vi "Initialize MeasurementLink Session.vi"(7 "remote connection options":T2, 8 "error in (no error)":errorcluster, 9 "initialize and close session behavior":T1, 10 "session initialization parameters":T3, 11 "instrument in":refnum<class "IInstrument.lvclass">) -> (0 "error out":errorcluster, 2 "session out":variant, 3 "instrument out":refnum<class "IInstrument.lvclass">)   [LabVIEW 2020, in "MeasurementLink Instrument.lvlib" / "IInstrument.lvclass"]
doc: "Creates a new session using the provided <b>session initialization parameters</b>. If the session represents a remote session, <b>initialize and close session behavior</b> determines whether creating the local session creates a new session on the server or attaches to an existing session on the server."
uses:
  IInstrument.lvclass
  Session Initialization Parameters.ctl
  Remote Connection Options.ctl
  Initialize and Close Session Behavior.ctl
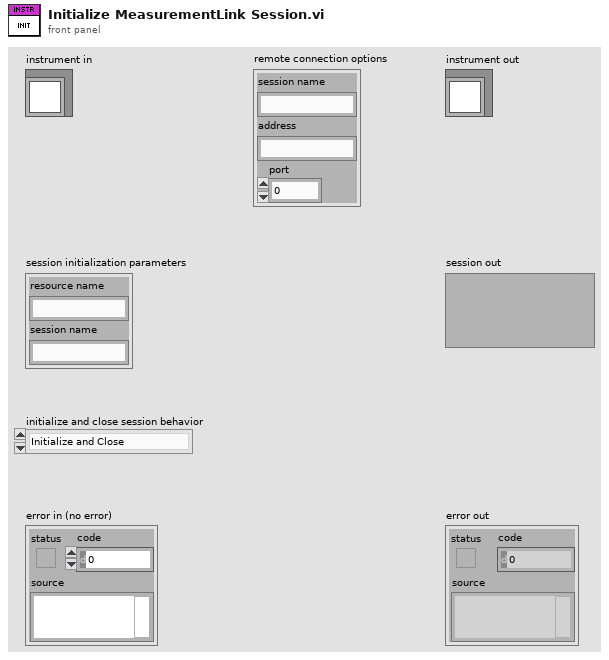
[diagram p1: front panel]
types:
  T1 = typedef "MeasurementLink Instrument.lvlib/IInstrument.lvclass/Initialize and Close Session Behavior.ctl" = enum16{"Initialize and Close", "Attach and Detach", "Initialize and Detach", "Attach and Close"}
  T2 = typedef "MeasurementLink Instrument.lvlib/IInstrument.lvclass/Remote Connection Options.ctl" = cluster{"session name":string, "address":string, "port":u32}
  T3 = typedef "MeasurementLink Instrument.lvlib/IInstrument.lvclass/Session Initialization Parameters.ctl" = cluster{"resource name":string, "session name":string}
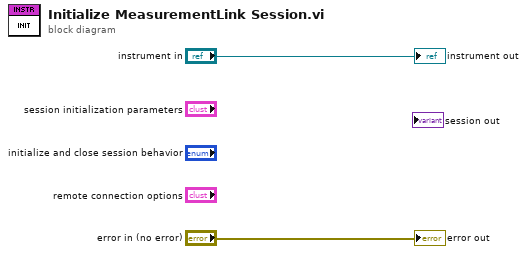
[diagram p0: block diagram]
diagram:
  "error out" <- "error in (no error)"
  "instrument out" <- "instrument in"
